vi "polar-view.vi"() -> ()   [LabVIEW 2017]
uses:
  <vilib>/Math Plots/2D Math Plots/2D Compass/2D Compass XCtrl/2D Compass.xctl
  <vilib>/Math Plots/2D Math Plots/2D Compass/2D Compass Datatype/Public/Plot Helper (Vector).vi
  <vilib>/Math Plots/2D Math Plots/2D Compass/2D Compass Datatype/2D Compass Datatype.lvclass
panel:
  out "Current value":dbl
  in  "stop":bool
  out "2D Compass":refnum<class "2D Plot Datatype.lvclass">[](xcontrol)
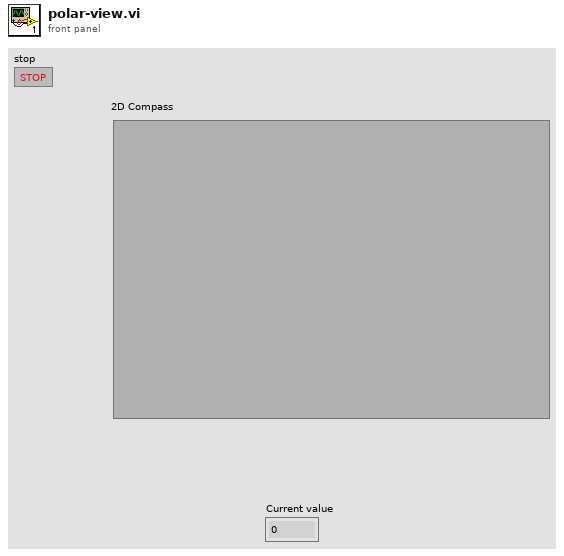
[diagram p1: front panel]
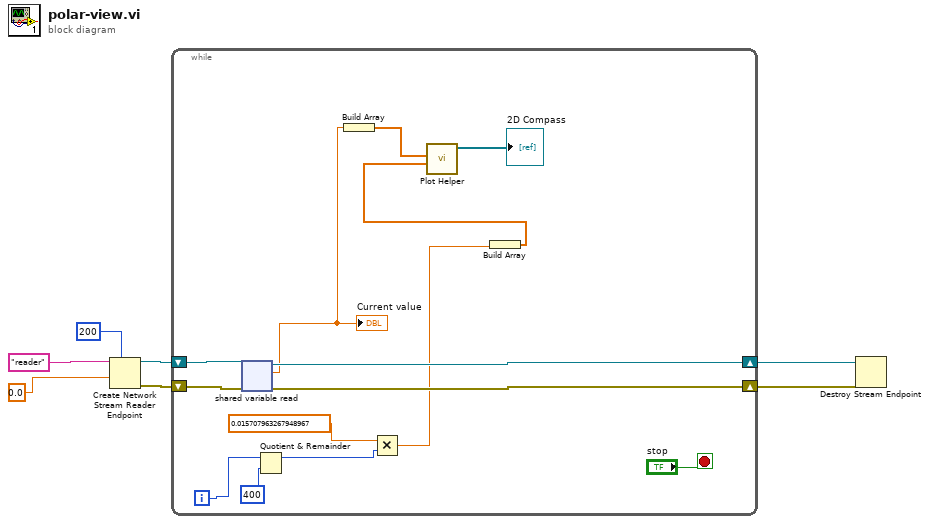
[diagram p0: block diagram]
diagram:
  n1 = Create Network Stream Reader Endpoint(7:200 ("reader buffer size"), 9:0.0, 11:"reader" ("reader name")) -> (0:w4:errorcluster, 3:w6:refnum<k21>)  [unwired: 4 in]
  n2 = while {
    shift-right: [w18] -> w5
    shift-left: w6 -> [w19]
    shift-right: [w16] -> w3
    shift-left: w4 -> [w17]
    i -> [w13]
    stop <- "stop" stop-if-true
    n3 = shared-variable-read(w19, w17) -> (w18:refnum<k21>, w16:errorcluster, w15:dbl)  [unwired: 1 in, 1 out]
    "Current value" <- w15
    n4 = Quotient & Remainder(x=w13, y=400) -> (x-y*floor(x/y)=w10:i32)  [unwired: 1 out]
    n5 = Build Array(w15) -> (w14:dbl[])
    n6 = Multiply(x=0.015707963267948967, y=w10) -> (x*y=w9:dbl)
    n7 = Build Array(w9) -> (w8:dbl[])
    n8 = call-poly <vilib>:"Plot Helper.vi"("radius vector"=w8, "theta vector"=w14) -> ("2D Plot Class Obj Array out"=→"2D Compass":refnum<class "2D Plot Datatype.lvclass">[])  [unwired: 2 in, 7 out]
  }
  n9 = Destroy Stream Endpoint(8:w3, 11:w5) -> ()  [unwired: 1 out]
